vi "Beta_Ver 1.1.vi"() -> ()   [LabVIEW 2015]
uses:
  <instrlib>/Keithley 622x LV 2009/Configure/Units/Typedefs/KE622x -- Voltage Meas Units.ctl
  <instrlib>/Keithley 622x LV 2009/Configure/2182 -A/Low Level/Typedefs/KE2182 -- Voltage Ranges.ctl
  <instrlib>/Keithley 622x LV 2009/Configure/2182 -A/Low Level/Typedefs/KE2182 -- Filter Type.ctl
  <instrlib>/Keithley 622x LV 2009/Configure/2182 -A/Low Level/Typedefs/KE2182 -- Filter Count.ctl
  <instrlib>/Keithley 622x LV 2009/Configure/2182 -A/Low Level/Typedefs/KE2182 -- Filter Window.ctl
  <instrlib>/Keithley 622x LV 2009/Configure/2182 -A/Low Level/Typedefs/KE2182 -- NPLCs.ctl
  <instrlib>/Keithley 622x LV 2009/Configure/Units/Typedefs/KE6221 -- PDelta Power Meas Type.ctl
  <instrlib>/Keithley 622x LV 2009/Configure/Delta PDelta DCon Modes/Typedefs/KE6221 -- PDelta Mode Params.ctl
  <instrlib>/Keithley 622x LV 2009/Configure/Delta PDelta DCon Modes/Low Level/Typedefs/KE622x -- Delta PDelta Mode High Level.ctl
  <instrlib>/Keithley 622x LV 2009/Configure/Delta PDelta DCon Modes/Low Level/Typedefs/KE622x -- Delta PDelta Mode Low Level.ctl
  <instrlib>/Keithley 622x LV 2009/Configure/Delta PDelta DCon Modes/Low Level/Typedefs/KE6221 -- PDelta Mode Pulse Width.ctl
  <instrlib>/Keithley 622x LV 2009/Configure/Delta PDelta DCon Modes/Low Level/Typedefs/KE6221 -- PDelta Mode Source Delay.ctl
  <instrlib>/Keithley 622x LV 2009/Configure/Delta PDelta DCon Modes/Low Level/Typedefs/KE622x -- Delta PDelta Mode Num Cycles Mode.ctl
  <instrlib>/Keithley 622x LV 2009/Configure/Delta PDelta DCon Modes/Low Level/Typedefs/KE622x -- Delta PDelta Mode Num Cycles.ctl
  <instrlib>/Keithley 622x LV 2009/Configure/Delta PDelta DCon Modes/Low Level/Typedefs/KE6221 -- PDelta Mode Ranging Mode.ctl
  <instrlib>/Keithley 622x LV 2009/Configure/Delta PDelta DCon Modes/Low Level/Typedefs/KE6221 -- PDelta Mode Num Low Meas.ctl
  <instrlib>/Keithley 622x LV 2009/Configure/Delta PDelta DCon Modes/Low Level/Typedefs/KE6221 -- PDelta Mode Pulse Period.ctl
  <instrlib>/Keithley 622x LV 2009/Configure/Format/Typedefs/KE622x -- Optional Meas Elements.ctl
  <instrlib>/Keithley 622x LV 2009/Configure/Trace Buf/Low Level/Typedefs/KE622x -- Trace Buf.ctl
  <instrlib>/Keithley 622x LV 2009/Configure/Delta PDelta DCon Modes/Low Level/Typedefs/KE622x -- Delta DCon Mode Delay.ctl
  <instrlib>/Keithley 622x LV 2009/Configure/Delta PDelta DCon Modes/Typedefs/KE622x -- Delta Mode Params.ctl
  <instrlib>/Keithley 622x LV 2009/Utility/Typedefs/KE622x -- Instrument Type.ctl
  <instrlib>/Keithley 622x LV 2009/Keithley 622x.lvlib
panel:
  out "COMMAND":string
  out "High Level (A)":T1=0.001 min=0.0 max=0.105 format="%.3e"
  out "Low Level (A)":T2=-0.001 min=-0.105 max=0.0 format="%.3e"
  out "Delay (s)":T3=0.002 min=0.001 max=9999.999 format="%.3f"
  out "Num Cycles Mode":T4
  out "Finite Count":T5=10 min=2 max=65536
  out "Abort On Compliance?":bool
  out "Cold Swithing Mode Enabled?":bool
  out "HI_L_COM":string
  out "LOW_L_COM":string
  out "COUN_COM":string
  out "COMP_COM":string
  out "COLD_COM":string
  out "DEL_COM":string
  out "FILE":refnum<file>
  out "Reading":sgl[](array[numeric])
  out "Trace Buf":T6 {"Average Voltage (V)" format="%.3p"; "Source Val (A)" format="%.3p"; "Timestamp (secs)" format="%.3f"; "Reading" format="%.7f"}
  in  "Meas Elements To Return":T7={"Timstamp?"=TRUE, "Reading Num?"=TRUE, "Source Value?"=FALSE, "Compliance?"=FALSE, "Average Voltage?"=FALSE}
  in  "stop":bool
  in  "Check For SCPI Errors? (T)":bool=TRUE
  in  "Power Meas Type":T8
  in  "2812 -A Params In":T14={"Auto Range?"=FALSE, "Man / Selected\nRange"=enum."10V", "Enable Digital\nFilter?"=FALSE, "Filter Type"=enum."Moving", "Filter Count"=10, "Filter\nWindow (%)"=0.01, "Enable Analog\nFilter?"=FALSE, "NPLCs"=5} {"Filter\nWindow (%)" min=0.0 max=10.0 step=0.01 format="%.2f"; "Filter Count" min=1 max=100; "NPLCs" min=1 max=10}
  in  "Measurement Units":T15
  in  "Measurements control":enum32{"PULSE", " DELTA"}(tab)
  in  "Pulsed Delta Mode Params In":T16={"High Level (A)"=0.001, "Low Level (A)"=0.0, "Pulse Width (s)"=0.00011, "Source Delay (s)"=1.6e-05, "Num Cycles Mode"=enum."Infinite", "Finite Count"=1, "Ranging Mode"=enum."Best", "Num Low Meas Per Cycle"=enum."2", "Pulse Period (Num PLCs)"=5, "Pulse Sweep Mode Enabled?"=FALSE} {"Pulse Period (Num PLCs)" min=5 max=999990; "Source Delay (s)" min=1.6e-05 max=0.011966 format="%.3p"; "Pulse Width (s)" min=5e-05 max=0.012 format="%.3p"; "Finite Count" min=2 max=65536; "Low Level (A)" min=-0.105 max=0.0 format="%.3p"; "High Level (A)" min=0.0 max=0.105 format="%.3p"}
  in  "Delta Mode Params In":T22={"High Level (A)"=0.001, "Low Level (A)"=-0.001, "Delay (s)"=0.002, "Num Cycles Mode"=enum."Finite Count", "Finite Count"=1, "Abort On\nCompliance?"=FALSE, "Cold Swithing\nMode Enabled?"=FALSE} {"Finite Count" min=1 max=65536; "Low Level (A)" min=-0.105 max=0.0 format="%.3p"; "High Level (A)" min=0.0 max=0.105 format="%.3p"; "Delay (s)" min=0.001 max=9999.999 format="%.3f"}
  in  "Comments":string
  in  "Folder \nPrename":string
  # "Keithley  6221 & 2182A Measurement System"
  # "FILE CONFIGURATION"
  # "PRE EXPERIMENT CONFIGS"
  # "*** NOTE:  \"Average Voltage\"\nis only available for Differential\nConductance measurements."
  # "*** NOTE:  \"Average Voltage\"\nis only available for Differential\nConductance measurements."
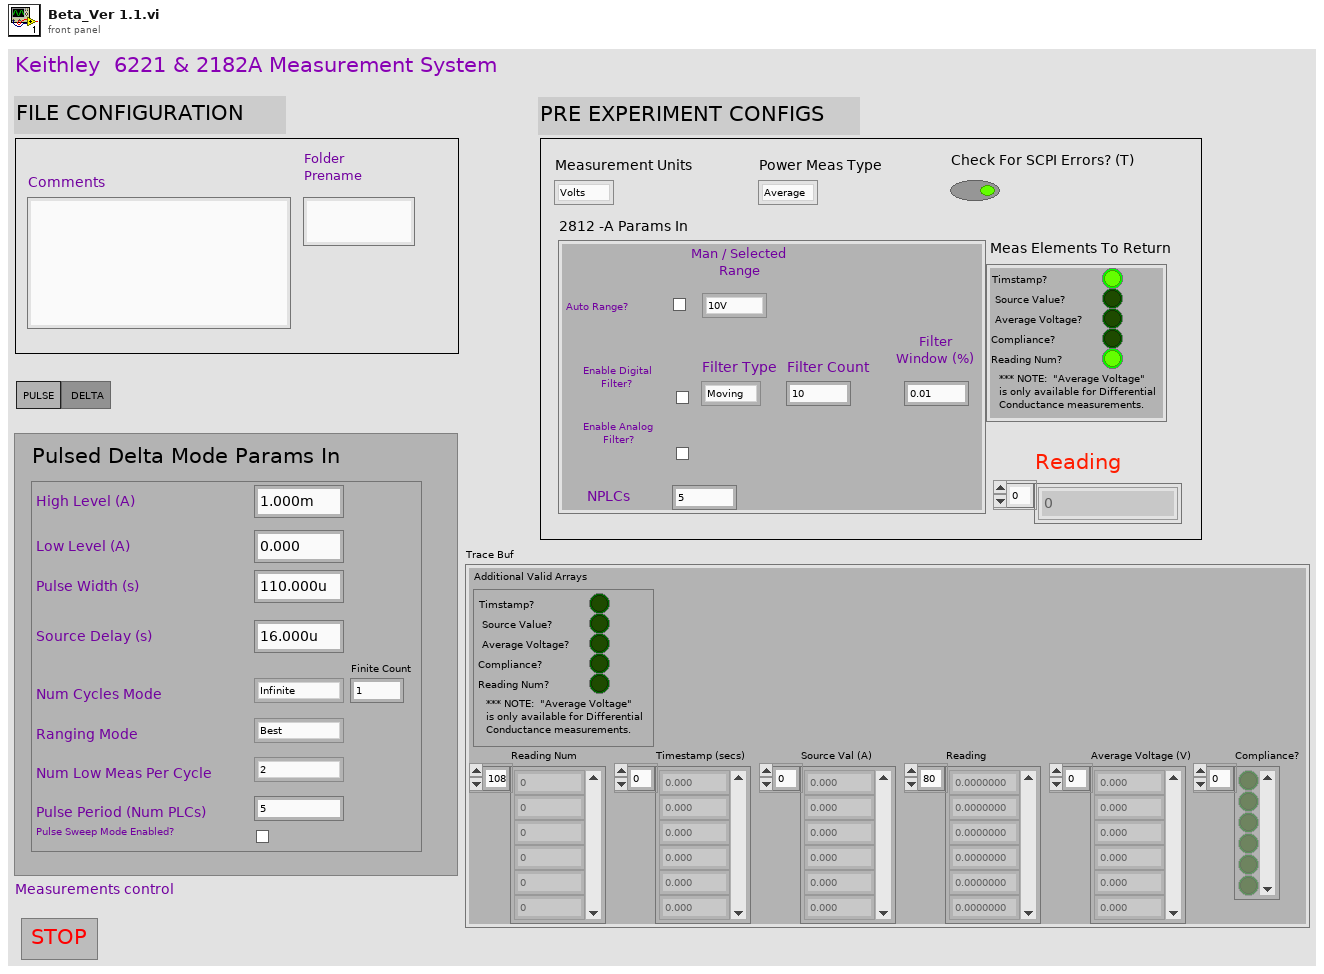
[diagram p1: front panel]
types:
  T1 = typedef "Keithley 622x.lvlib/KE622x -- Delta PDelta Mode High Level.ctl" = dbl
  T2 = typedef "Keithley 622x.lvlib/KE622x -- Delta PDelta Mode Low Level.ctl" = dbl
  T3 = typedef "Keithley 622x.lvlib/KE622x -- Delta DCon Mode Delay.ctl" = dbl
  T4 = typedef "Keithley 622x.lvlib/KE622x -- Delta PDelta Mode Num Cycles Mode.ctl" = enum16{"Finite Count", "Infinite"}
  T5 = typedef "Keithley 622x.lvlib/KE622x -- Delta PDelta Mode Num Cycles.ctl" = u32
  T6 = typedef "Keithley 622x.lvlib/KE622x -- Trace Buf.ctl" = cluster{"Additional Valid Arrays":T7, "Reading Num":u32[], "Timestamp (secs)":sgl[], "Source Val (A)":sgl[], "Reading":sgl[], "Average Voltage (V)":sgl[], "Compliance?":bool[]}
  T7 = typedef "Keithley 622x.lvlib/KE622x -- Optional Meas Elements.ctl" = cluster{"Timstamp?":bool, "Reading Num?":bool, "Source Value?":bool, "Compliance?":bool, "Average Voltage?":bool}
  T8 = typedef "Keithley 622x.lvlib/KE6221 -- PDelta Power Meas Type.ctl" = enum16{"Average", "Peak"}
  T9 = typedef "Keithley 622x.lvlib/KE2182 -- Voltage Ranges.ctl" = enum16{"10mV", "100mV", "1V", "10V", "100V"}
  T10 = typedef "Keithley 622x.lvlib/KE2182 -- Filter Type.ctl" = enum16{"Moving", "Repeat"}
  T11 = typedef "Keithley 622x.lvlib/KE2182 -- Filter Count.ctl" = u32
  T12 = typedef "Keithley 622x.lvlib/KE2182 -- Filter Window.ctl" = dbl
  T13 = typedef "Keithley 622x.lvlib/KE2182 -- NPLCs.ctl" = u32
  T14 = cluster{"Auto Range?":bool, "Man / Selected\nRange":T9, "Enable Digital\nFilter?":bool, "Filter Type":T10, "Filter Count":T11, "Filter\nWindow (%)":T12, "Enable Analog\nFilter?":bool, "NPLCs":T13}
  T15 = typedef "Keithley 622x.lvlib/KE622x -- Voltage Meas Units.ctl" = enum16{"Volts", "Ohms", "Watts", "Siemens"}
  T16 = typedef "Keithley 622x.lvlib/KE6221 -- PDelta Mode Params.ctl" = cluster{"High Level (A)":T1, "Low Level (A)":T2, "Pulse Width (s)":T17, "Source Delay (s)":T18, "Num Cycles Mode":T4, "Finite Count":T5, "Ranging Mode":T19, "Num Low Meas Per Cycle":T20, "Pulse Period (Num PLCs)":T21, "Pulse Sweep Mode Enabled?":bool}
  T17 = typedef "Keithley 622x.lvlib/KE6221 -- PDelta Mode Pulse Width.ctl" = dbl
  T18 = typedef "Keithley 622x.lvlib/KE6221 -- PDelta Mode Source Delay.ctl" = dbl
  T19 = typedef "Keithley 622x.lvlib/KE6221 -- PDelta Mode Ranging Mode.ctl" = enum16{"Best", "Fixed"}
  T20 = typedef "Keithley 622x.lvlib/KE6221 -- PDelta Mode Num Low Meas.ctl" = enum16{"1", "2"}
  T21 = typedef "Keithley 622x.lvlib/KE6221 -- PDelta Mode Pulse Period.ctl" = u32
  T22 = typedef "Keithley 622x.lvlib/KE622x -- Delta Mode Params.ctl" = cluster{"High Level (A)":T1, "Low Level (A)":T2, "Delay (s)":T3, "Num Cycles Mode":T4, "Finite Count":T5, "Abort On\nCompliance?":bool, "Cold Swithing\nMode Enabled?":bool}
  T23 = typedef "Keithley 622x.lvlib/KE622x -- Instrument Type.ctl" = enum16{"KE6220", "KE6221"}
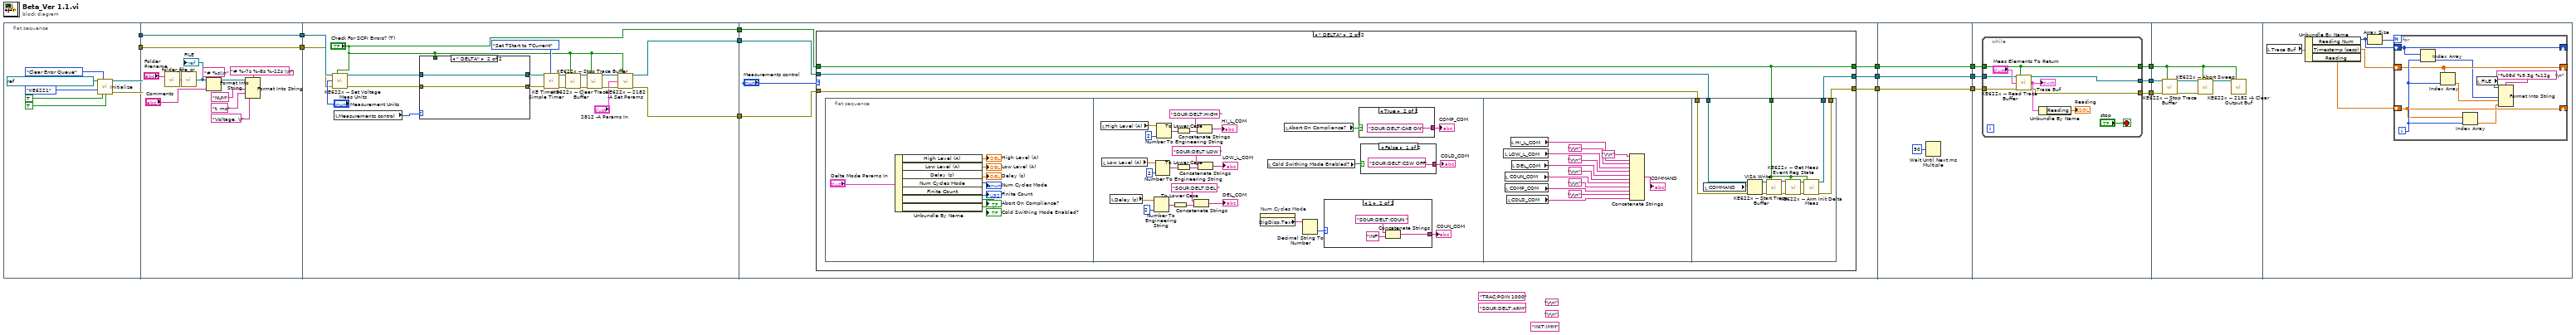
[diagram p0: block diagram]
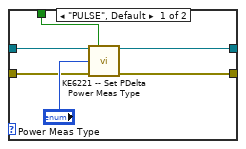
[diagram p2: hidden frame]
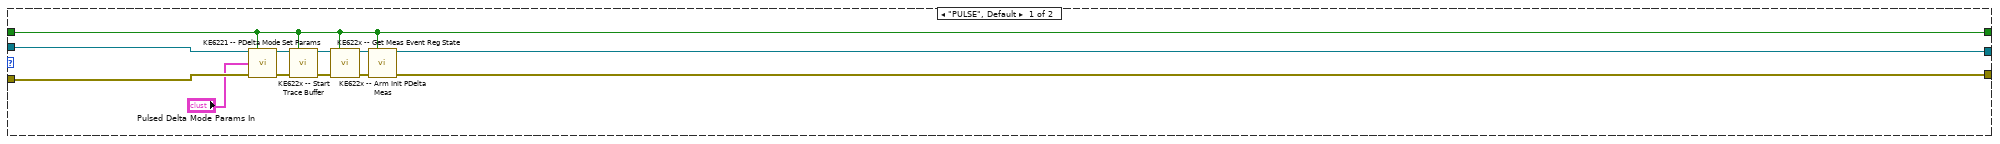
[diagram p3: hidden frame]
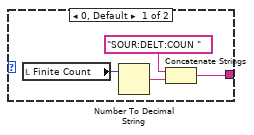
[diagram p4: hidden frame]
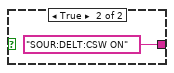
[diagram p5: hidden frame]
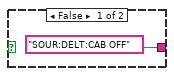
[diagram p6: hidden frame]
diagram:
  (unwired) "INIT:IMM" ("string")
  (unwired) "SOUR:DELT:ARM" ("string")
  (unwired) "TRAC:POIN 1000" ("string")
  (unwired) "\r\n"
  (unwired) "\r\n"
  n1 = flat-sequence {
    tunnel: [w18] -> w10
    tunnel: [w17] -> w8
    tunnel: w10 -> [w35]
    tunnel: [w35] -> w9
    tunnel: w8 -> [w34]
    tunnel: [w34] -> w7
    tunnel: w9 -> [w53]
    tunnel: w7 -> [w52]
    tunnel: [w43] -> w16
    tunnel: [w42] -> w15
    tunnel: ["Check For SCPI Errors? (T)"] -> w14
    tunnel: w16 -> [w67]
    tunnel: w15 -> [w68]
    tunnel: w14 -> [w66]
    tunnel: [w65] -> w6
    tunnel: [w64] -> w4
    tunnel: [w63] -> w2
    tunnel: w6 -> [w159]
    tunnel: [w159] -> w5
    tunnel: w4 -> [w158]
    tunnel: [w158] -> w3
    tunnel: w2 -> [w157]
    tunnel: [w157] -> w1
    tunnel: w5 -> [w165]
    tunnel: w3 -> [w164]
    tunnel: w1 -> [w163]
    tunnel: [w162] -> w13
    tunnel: [w161] -> w12
    tunnel: [w160] -> w11
    tunnel: w13 -> [w178]
    tunnel: w12 -> [w177]
    tunnel: w11 -> [w175]
    frame #0 {
      n2 = call <instrlib>:"Initialize.vi"("VISA resource name"=refnum<visa-resource-name> "DC_AC_Current_Source_6221", "Error Queue Option"=enum16{"Clear Error Queue", "Error Query"}."Clear Error Queue", "Instrument Type"=KE622x_--_Instrument_Type."KE6221", "ID Query? (T)"=TRUE, "Reset? (T)"=TRUE) -> ("VISA resource name out"=w18:refnum<visa-resource-name>, "error out"=w17:errorcluster)  [unwired: 9 in]
    }
    frame #1 {
      n3 = call "folder_cr.vi"("Name"="Folder \nPrename") -> ("String"=w26:string)
      n4 = call "file_cr.vi"("String"=w26) -> ("refnum out"=w24:refnum<file>)
      "FILE" <- w24
      n5 = Format Into String(format string="# %s\\n", initial string=w24, "Comments") -> (resulting string=w31:refnum<file>)  [unwired: 1 in, 1 out]
      n6 = Format Into String(format string="# %-7s %-8s %-12s \\n", initial string=w31, "NUM" ("input 1"), "t, ms" ("input 2"), "Voltage, V" ("input 3")) -> ()  [unwired: 1 in, 2 out]
    }
    frame #2 {
      n7 = call <instrlib>:"KE622x -- Set Voltage Meas Units.vi"("Resource In"=w53, "Check For SCPI Errors? (T)"="Check For SCPI Errors? (T)", "Voltage Meas Units"="Measurement Units", "error in (no error)"=w52) -> ("Resource Out (dupl)"=w39:refnum<visa-resource-name>, "error out"=w38:errorcluster)  [unwired: 10 in]
      n8 = local read "Measurements control"() -> (w41:enum32{"PULSE", " DELTA"})
      n9 = case shown="\" DELTA\"" w41 {
        tunnel: "Check For SCPI Errors? (T)" -> [w59 _]
        tunnel: w39 -> [w58 w62]
        tunnel: w38 -> [w57 w61]
        tunnel: [w56 w62] -> w37
        tunnel: [w55 w61] -> w36
        frame "PULSE", Default {
          n10 = call <instrlib>:"KE6221 -- Set PDelta Power Meas Type.vi"("6221 Resource In"=w58, "Check For SCPI Errors? (T)"=w59, "Power Meas Type"="Power Meas Type", "error in (no error)"=w57) -> ("6221 Resource Out (dupl)"=w56:refnum<visa-resource-name>, "error out"=w55:errorcluster)  [unwired: 10 in]
        }
        frame " DELTA" {
        }
      }
      n11 = call <instrlib>:"KE Timer -- Simple Timer.vi"("Resource In"=w37, "error in (no error)"=w36, "Action"=enum16{"Set TStart to TCurrent", "Get Deltas"}."Set TStart to TCurrent") -> ("Resource Out (dupl)"=w50:refnum<visa-resource-name>, "error out (dupl)"=w49:errorcluster)  [unwired: 7 in, 8 out]
      n12 = call <instrlib>:"KE622x -- Stop Trace Buffer.vi"("Resource In"=w50, "Check For SCPI Errors? (T)"="Check For SCPI Errors? (T)", "error in (no error)"=w49) -> ("Resource Out (dupl)"=w48:refnum<visa-resource-name>, "error out"=w47:errorcluster)  [unwired: 11 in]
      n13 = call <instrlib>:"KE622x -- Clear Trace Buffer.vi"("Resource In"=w48, "Check For SCPI Errors? (T)"="Check For SCPI Errors? (T)", "error in (no error)"=w47) -> ("Resource Out (dupl)"=w46:refnum<visa-resource-name>, "error out"=w45:errorcluster)  [unwired: 11 in]
      n14 = call <instrlib>:"KE622x -- 2182 -A Set Params.vi"("622x Resource In"=w46, "Check For SCPI Errors? (T)"="Check For SCPI Errors? (T)", "2812 -A Params In"="2812 -A Params In", "error in (no error)"=w45) -> ("622x Resource Out (dupl)"=w43:refnum<visa-resource-name>, "error out"=w42:errorcluster)  [unwired: 9 in, 1 out]
    }
    frame #3 {
      n15 = case shown="\" DELTA\"" "Measurements control" {
        tunnel: w68 -> [w80 w85]
        tunnel: w67 -> [w81 w86]
        tunnel: w66 -> [w70 w84]
        tunnel: [w72 w83] -> w65
        tunnel: [w71 w82] -> w64
        tunnel: [w70 w84] -> w63
        frame "PULSE", Default {
          n16 = call <instrlib>:"KE6221 -- PDelta Mode Set Params.vi"("6221 Resource In"=w81, "Check For SCPI Errors? (T)"=w70, "Pulsed Delta Mode Params In"="Pulsed Delta Mode Params In", "error in (no error)"=w80) -> ("6221 Resource Out (dupl)"=w78:refnum<visa-resource-name>, "error out"=w77:errorcluster)  [unwired: 9 in, 1 out]
          n17 = call <instrlib>:"KE622x -- Start Trace Buffer.vi"("Resource In"=w78, "Check For SCPI Errors? (T)"=w70, "error in (no error)"=w77) -> ("Resource Out (dupl)"=w76:refnum<visa-resource-name>, "error out"=w75:errorcluster)  [unwired: 11 in]
          n18 = call <instrlib>:"KE622x -- Get Meas Event Reg State.vi"("VISA Resource In"=w76, "Error Query (T)?"=w70, "error in (no error)"=w75) -> ("VISA Resource Out (dupl)"=w74:refnum<visa-resource-name>, "error out"=w73:errorcluster)  [unwired: 10 in, 1 out]
          n19 = call <instrlib>:"KE622x -- Arm Init PDelta Meas.vi"("Resource In"=w74, "Check For SCPI Errors? (T)"=w70, "error in (no error)"=w73) -> ("Resource Out (dupl)"=w72:refnum<visa-resource-name>, "error out"=w71:errorcluster)  [unwired: 11 in]
        }
        frame " DELTA" {
          n20 = flat-sequence {
            tunnel: w86 -> [w155]
            tunnel: w85 -> [w154]
            tunnel: w84 -> [w146]
            tunnel: [w145] -> w83
            tunnel: [w144] -> w82
            frame #0 {
              n21 = Unbundle By Name("Delta Mode Params In") -> ("High Level (A)"=→"High Level (A)":T1, "Low Level (A)"=→"Low Level (A)":T2, "Delay (s)"=→"Delay (s)":T3, "Num Cycles Mode"=→"Num Cycles Mode":T4, "Finite Count"=→"Finite Count":T5, "Abort On\nCompliance?"=→"Abort On Compliance?":bool, "Cold Swithing\nMode Enabled?"=→"Cold Swithing Mode Enabled?":bool)
            }
            frame #1 {
              n22 = local read "High Level (A)"() -> (w118:T1)
              n23 = local read "Low Level (A)"() -> (w117:T2)
              n24 = local read "Delay (s)"() -> (w114:T3)
              n25 = Number To Engineering String(2:i16 2 ("precision (6)"), 4:w114) -> (0:w103:string)  [unwired: 2 in]
              n26 = Number To Engineering String(2:i16 2 ("precision (6)"), 4:w117) -> (0:w105:string)  [unwired: 2 in]
              n27 = Number To Engineering String(2:i16 2 ("precision (6)"), 4:w118) -> (0:w106:string)  [unwired: 2 in]
              n28 = To Lower Case(string=w103) -> (all lower case string=w102:string)
              n29 = To Lower Case(string=w106) -> (all lower case string=w107:string)
              n30 = To Lower Case(string=w105) -> (all lower case string=w104:string)
              n31 = Concatenate Strings("SOUR:DELT:DEL " ("string"), w102) -> (→"DEL_COM":string)
              n32 = Concatenate Strings("SOUR:DELT:HIGH " ("string"), w107) -> (→"HI_L_COM":string)
              n33 = Concatenate Strings("SOUR:DELT:LOW " ("string"), w104) -> (→"LOW_L_COM":string)
              n34 = property on="Num Cycles Mode" class="Enum (strict)"() -> ("DigDisp.Text"=w97:string)  [unwired: 2 in, 2 out]
              n35 = local read "Cold Swithing Mode Enabled?"() -> (w98:bool)
              n36 = local read "Abort On Compliance?"() -> (w99:bool)
              n37 = Decimal String To Number(string=w97) -> (number=w96:i32)  [unwired: 2 in, 1 out]
              n38 = case shown="1" w96 {
                tunnel: [w120 w124] -> w95
                frame 0, Default {
                  n39 = local read "Finite Count"() -> (w122:T5)
                  n40 = Number To Decimal String(number=w122) -> (decimal integer string=w121:string)  [unwired: 1 in]
                  n41 = Concatenate Strings("SOUR:DELT:COUN " ("string"), w121) -> (w120:string)
                }
                frame 1 {
                  n42 = Concatenate Strings("SOUR:DELT:COUN " ("string"), "INF" ("string")) -> (w124:string)
                }
              }
              "COUN_COM" <- w95
              n43 = case shown="True" w99 {
                tunnel: ["SOUR:DELT:CAB OFF" ("string") "SOUR:DELT:CAB ON" ("string")] -> w101
                frame False {
                }
                frame True {
                }
              }
              "COMP_COM" <- w101
              n44 = case shown="False" w98 {
                tunnel: ["SOUR:DELT:CSW OFF" ("string") "SOUR:DELT:CSW ON" ("string")] -> w100
                frame False {
                }
                frame True {
                }
              }
              "COLD_COM" <- w100
            }
            frame #2 {
              n45 = local read "LOW_L_COM"() -> (w139:string)
              n46 = local read "COUN_COM"() -> (w141:string)
              n47 = local read "COMP_COM"() -> (w142:string)
              n48 = local read "COLD_COM"() -> (w143:string)
              n49 = local read "HI_L_COM"() -> (w138:string)
              n50 = local read "DEL_COM"() -> (w140:string)
              n51 = Concatenate Strings("\r\n", w138, "\r\n", w139, "\r\n", w140, "\r\n", w141, "\r\n", w142, "\r\n", w143) -> (→"COMMAND":string)
            }
            frame #3 {
              n52 = local read "COMMAND"() -> (w153:string)
              n53 = VISA Write(VISA resource name=w155, write buffer=w153, error in (no error)=w154) -> (VISA resource name out=w151:refnum<visa-resource-name>, error out=w152:errorcluster)  [unwired: 1 out]
              n54 = call <instrlib>:"KE622x -- Start Trace Buffer.vi"("Resource In"=w151, "Check For SCPI Errors? (T)"=w146, "error in (no error)"=w152) -> ("Resource Out (dupl)"=w150:refnum<visa-resource-name>, "error out"=w149:errorcluster)  [unwired: 11 in]
              n55 = call <instrlib>:"KE622x -- Get Meas Event Reg State.vi"("VISA Resource In"=w150, "Error Query (T)?"=w146, "error in (no error)"=w149) -> ("VISA Resource Out (dupl)"=w147:refnum<visa-resource-name>, "error out"=w148:errorcluster)  [unwired: 10 in, 1 out]
              n56 = call <instrlib>:"KE622x -- Arm Init Delta Meas.vi"("Resource In"=w147, "Check For SCPI Errors? (T)"=w146, "error in (no error)"=w148) -> ("Resource Out (dupl)"=w145:refnum<visa-resource-name>, "error out"=w144:errorcluster)  [unwired: 11 in]
            }
          }
        }
      }
    }
    frame #4 {
      n57 = Wait Until Next ms Multiple(millisecond multiple=u32 50) -> ()  [unwired: 1 out]
    }
    frame #5 {
      n58 = while {
        tunnel: w165 -> [w171]
        tunnel: w164 -> [w172]
        tunnel: w163 -> [w170]
        tunnel: [w170] -> w162
        tunnel: [w169] -> w161
        tunnel: [w168] -> w160
        stop <- "stop" stop-if-true
        n59 = call <instrlib>:"KE622x -- Read Trace Buffer.vi"("Resource In"=w171, "Check For SCPI Errors? (T)"=w170, "Meas Elements To Return"="Meas Elements To Return", "error in (no error)"=w172) -> ("Resource Out (dupl)"=w169:refnum<visa-resource-name>, "Trace Buf"=w167:T6, "error out"=w168:errorcluster)  [unwired: 9 in]
        "Trace Buf" <- w167
        n60 = Unbundle By Name(w167) -> ("Reading"=→"Reading":sgl[])
      }
    }
    frame #6 {
      n61 = call <instrlib>:"KE622x -- Stop Trace Buffer.vi"("Resource In"=w177, "Check For SCPI Errors? (T)"=w178, "error in (no error)"=w175) -> ("Resource Out (dupl)"=w180:refnum<visa-resource-name>, "error out"=w176:errorcluster)  [unwired: 11 in]
      n62 = call <instrlib>:"KE622x -- Abort Sweep.vi"("Resource In"=w180, "Check For SCPI Errors? (T)"=w178, "error in (no error)"=w176) -> ("Resource Out (dupl)"=w179:refnum<visa-resource-name>)  [unwired: 11 in, 1 out]
      n63 = call <instrlib>:"KE622x -- 2182 -A Clear Output Buf.vi"("622x Resource In"=w179, "Check For SCPI Errors? (T)"=w178) -> ()  [unwired: 11 in, 3 out]
    }
    frame #7 {
      n64 = local read "Trace Buf"() -> (w185:T6)
      n65 = Unbundle By Name(w185) -> ("Reading Num"=w181:u32[], "Timestamp (secs)"=w183:sgl[], "Reading"=w182:sgl[])
      n66 = Array Size(array=w181) -> (size(s)=w184:i32)
      n67 = for {
        N: w184 -> [_]
        shift-right: [w193] -> _
        shift-left: w181 -> [w193]
        shift-right: [w192] -> _
        shift-left: w183 -> [w192]
        shift-right: [w191] -> _
        shift-left: w182 -> [w191]
        i -> [w194]
        n68 = Index Array(array=w193, index=w194) -> (element=w188:u32)
        n69 = Index Array(array=w192, index=w194) -> (element=w187:sgl)
        n70 = Index Array(array=w191, index=w194) -> (element=w186:sgl)
        n71 = local read "FILE"() -> (w190:refnum<file>)
        n72 = Format Into String(format string="%08d %9.3g %12g   \\n", initial string=w190, w188, w187, w186) -> ()  [unwired: 1 in, 2 out]
      }
    }
  }
